vi "Main.vi"   [LabVIEW 2022 SP3, in "TouchControl.lvlib"]
uses:
  TouchControl.lvlib
  TouchControl/TouchControl.lvclass
types:
  T1 = enum32{"Invalid", "Standard", "Closed", "Hidden", "Minimized", "Maximized"}
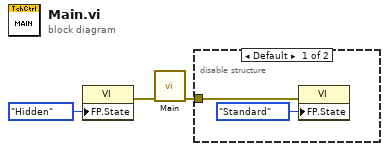
[diagram p0: block diagram]
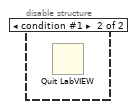
[diagram p2: hidden frame]
diagram:
  n1 = property class="VI"("FP.State"=T1."Hidden" ("Front Panel Window:State")) -> (error out=w3:errorcluster)  [unwired: 2 in, 1 out]
  n2 = call "Main.vi"("error in (no error)"=w3) -> ("error out"=w1:errorcluster)  [unwired: 10 in]
  n3 = disable-structure shown="Default" {
    disable-tunnel: w1 -> [w5 _]
    frame condition #0 (active) {
      n4 = property class="VI"(error in=w5, "FP.State"=T1."Standard" ("Front Panel Window:State")) -> ()  [unwired: 1 in, 2 out]
    }
    frame condition #1 {
      n5 = Quit LabVIEW() -> ()  [unwired: 1 in]
    }
  }
